vi "LV SPECTRUM START.vi"(0 "min":u32, 1 "max":u32=65535, 2 "limitmode":string(combo)="freerun", 3 "limit":u32, 5 "rebin":u32, 7 "Spectrum name":string, 9 "Handle In":T2) -> (10 "Handle Out":T1)   [LabVIEW 2021]
uses:
  SciSDK_Labview.lvlib
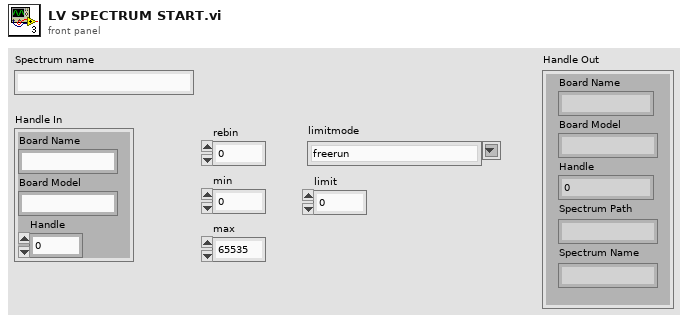
[diagram p1: front panel]
types:
  T1 = cluster{"Board Name":string, "Board Model":string, "Handle":u64, "Spectrum Path":string, "Spectrum Name":string}
  T2 = cluster{"Board Name":string, "Board Model":string, "Handle":u64}
  T3 = cluster{"Board Name":string, "Board Model":string, "Handle":u64, string, "Spectrum name":string}
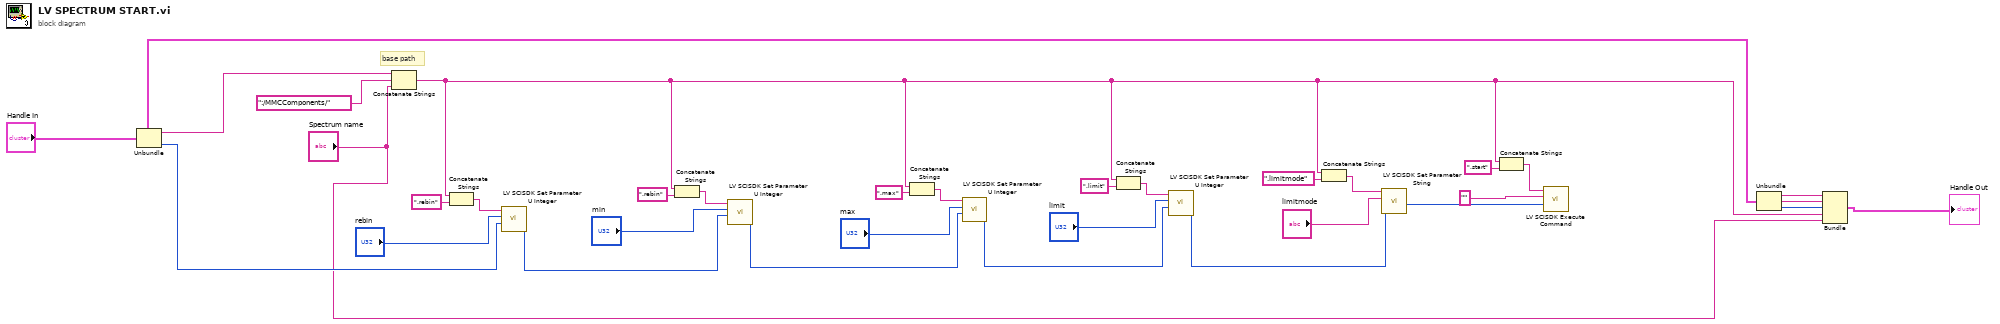
[diagram p0: block diagram]
diagram:
  # "base path"
  n1 = Unbundle("Handle In") -> ("Board Name"=w32:string, "Handle"=w28:u64)  [unwired: 1 out]
  n2 = Concatenate Strings(w32, ":/MMCComponents/" ("string"), "Spectrum name") -> (w1:string)
  n3 = Concatenate Strings(w1, ".rebin" ("string")) -> (w30:string)
  n4 = call "LV SCISDK Set Parameter U Integer.vi"("handle"=w28, "value"="rebin", "Path"=w30) -> ("handle out"=w21:u64)  [unwired: 6 in, 2 out]
  n5 = Concatenate Strings(w1, ".rebin" ("string")) -> (w26:string)
  n6 = call "LV SCISDK Set Parameter U Integer.vi"("handle"=w21, "value"="min", "Path"=w26) -> ("handle out"=w19:u64)  [unwired: 6 in, 2 out]
  n7 = Concatenate Strings(w1, ".max" ("string")) -> (w24:string)
  n8 = call "LV SCISDK Set Parameter U Integer.vi"("handle"=w19, "value"="max", "Path"=w24) -> ("handle out"=w17:u64)  [unwired: 6 in, 2 out]
  n9 = Concatenate Strings(w1, ".limit" ("string")) -> (w22:string)
  n10 = call "LV SCISDK Set Parameter U Integer.vi"("handle"=w17, "value"="limit", "Path"=w22) -> ("handle out"=w15:u64)  [unwired: 6 in, 2 out]
  n11 = Concatenate Strings(w1, ".limitmode" ("string")) -> (w12:string)
  n12 = call "LV SCISDK Set Parameter String.vi"("handle"=w15, "value"="limitmode", "Path"=w12) -> ("handle out"=w5:u64)  [unwired: 6 in, 2 out]
  n13 = Concatenate Strings(w1, ".start" ("string")) -> (w2:string)
  n14 = call "LV SCISDK Execute Command.vi"("handle"=w5, "value"="", "Path"=w2) -> ()  [unwired: 6 in, 3 out]
  n15 = Unbundle("Handle In") -> ("Board Name"=w10:string, "Board Model"=w9:string, "Handle"=w8:u64)
  n16 = Bundle("Board Name"=w10, "Board Model"=w9, "Handle"=w8, w1, "Spectrum name"="Spectrum name") -> (→"Handle Out":T3)  [unwired: 1 in]
